vi "CC FG Recent Images.vi"(8 "error in (no error)":errorcluster, 10 "Write":bool, 11 "Recent Images":T1[](array[typedef]) {"Detector #" items=["None", "YJ", "HK"]}) -> (0 "error out":errorcluster, 3 "Recent Images out":T1[](array[typedef]) {"Detector #" items=["None", "YJ", "HK"]})   [LabVIEW 2024]
uses:
  Subsystems/SS cluster New Image Data.ctl
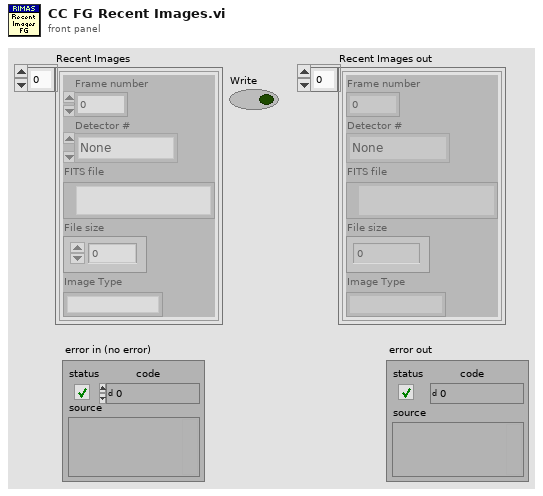
[diagram p1: front panel]
types:
  T1 = typedef "SS cluster New Image Data.ctl" = cluster{"Frame number":i32, "Detector #":u16, "FITS file":path, "File size":i64, "Image Type":string}
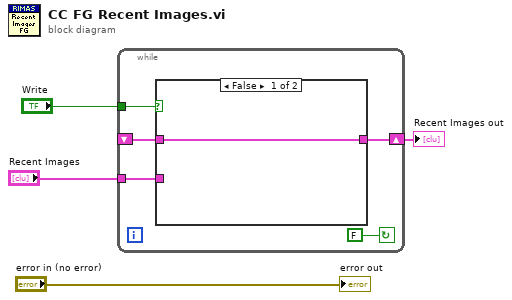
[diagram p0: block diagram]
diagram:
  n1 = while {
    tunnel: "Write" -> [w8]
    tunnel: "Recent Images" -> [w7]
    shift-right: [w6] -> w1
    shift-left: _ -> [w5]
    stop <- FALSE continue-if-true
    n2 = case shown="False" w8 {
      tunnel: w7 -> [_ w11]
      tunnel: [w10 w11] -> w6
      tunnel: w5 -> [w10 _]
      frame False {
      }
      frame True {
      }
    }
  }
  "Recent Images out" <- w1
  "error out" <- "error in (no error)"
